vi "Image_Crop_to_Object.vi"(8 "Particle Measurements":dbl[][](array[numeric])=[[57.0, 126.0, 60.0, 134.0, 14.0], [248.0, 156.0, 341.0, 306.0, 6231.0], [31.0, 193.0, 32.0, 194.0, 1.0], [324.0, 201.0, 327.0, 209.0, 15.0], [350.0, 252.0, 359.0, 273.0, 108.0], [55.0, 573.0, 56.0, 576.0, 3.0]]) -> (0 "ROI descriptor":T1={"Global Rectangle"=[233, 141, 356, 321], "Contours"=[{"ID"=enum."External", "Type"=3, "Coordinates"=[233, 141, 356, 321]}]}, 3 "Object detected":bool=TRUE)   [LabVIEW 2019]
panel:
  out "output array":i32[](array[numeric])
  out "Max area detected":dbl=6231.0
  in  "Crop trim":dbl[](array[numeric])=[-15.0, -15.0, 15.0, 15.0]
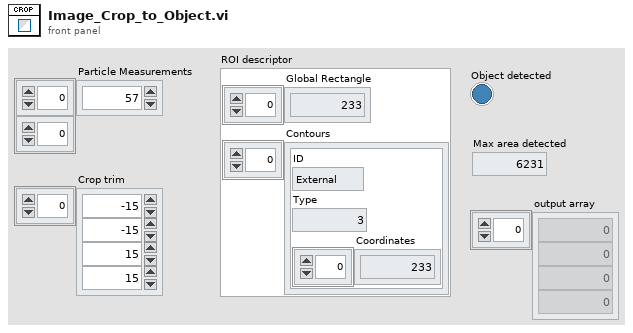
[diagram p1: front panel]
types:
  T1 = cluster{"Global Rectangle":i32[], "Contours":cluster{"ID":enum32{"External", "Internal"}, "Type":u32, "Coordinates":i32[]}[]}
  T2 = cluster{"ID":enum32{"External", "Internal"}, "Type":u32, "Coordinates":i32[]}[]
  T3 = cluster{"ID":enum32{"External", "Internal"}, "Type":u32, "Coordinates":i32[]}
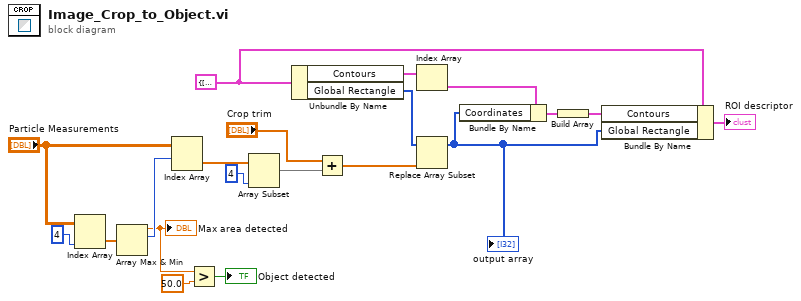
[diagram p0: block diagram]
diagram:
  w1 = T1 {"Global Rectangle"=[106, 29, 356, 265], "Contours"=[{"ID"=enum."External", "Type"=3, "Coordinates"=[106, 29, 356, 265]}]} ("Crop to object")
  n1 = Index Array(array="Particle Measurements", index (col)=4 ("index (row)")) -> (element=w8:dbl[])  [unwired: 1 in]
  n2 = Array Max & Min(array=w8) -> (max value=w4:dbl, max index (indices)=w5:i32)  [unwired: 2 out]
  "Max area detected" <- w4
  n3 = Index Array(array="Particle Measurements", index (row)=w5) -> (element=w12:dbl[])  [unwired: 1 in]
  n4 = Greater?(x=w4, y=50.0) -> (0:→"Object detected":bool)
  n5 = Array Subset(array=w12, length=4) -> (w11:dbl[])  [unwired: 1 in]
  n6 = Unbundle By Name(w1) -> ("Contours"=w19:T2, "Global Rectangle"=w20:i32[])
  n7 = Add(x="Crop trim", y=w11) -> (x+y=w9:dbl[])
  n8 = Index Array(array=w19) -> (element=w18:T3)  [unwired: 1 in]
  n9 = Replace Array Subset(array=w20, new element=w9) -> (w17:i32[])  [unwired: 1 in]
  "output array" <- w17
  n10 = Bundle By Name(cluster=w18, "Coordinates"=w17) -> (w16:T3)
  n11 = Build Array(w16) -> (w15:T2)
  n12 = Bundle By Name(cluster=w1, "Contours"=w15, "Global Rectangle"=w17) -> (→"ROI descriptor":T1)
